vi "auto_direct_attack_v2.vi"() -> ()   [LabVIEW 2012, in "MainProject.lvrbt"]
uses:
  MainProject.lvrbt
  <vilib>/NXT/Hardware/Plugins/Tetrix DC Motor/TetrixDCMotorAddress.ctl
  Drivers/AutoControlDirectAttackV2.ctl
  Drivers/LineDetectCtl.ctl
  Drivers/AutoDriverControl.ctl
  <vilib>/NXT/HiTechnic/HiTechnic Controls/HiTechnic Port.ctl
  <vilib>/NXT/Block Support/NXT_InputPort.ctl
  Drivers/LineCounterControl.ctl
  FTC 2012 - 2013/Controls/SpeedControl.ctl
  <vilib>/NXT/NXTIO Xnodes/NXTIONodeSubVIs/TETRIX IO Check Battery.vi
  <vilib>/NXT/Dual Mode Library/Waits/Wait_Num(msec).vi
  <vilib>/NXT/NXTIO Xnodes/NXTIONodeSubVIs/TETRIX IO Stop DC Motors.vi
  <vilib>/NXT/Dual Mode Library/Sound/Tone.vi
  <vilib>/NXT/Dual Mode Library/Display/drawNumber.vi
  <vilib>/NXT/Subs/LVHSConnector.ctl
  <vilib>/NXT/NXTIO Xnodes/AddressXNode/NXTIOAddress.xnode
  <vilib>/NXT/NXTIO Xnodes/NXTIOXNode/NXTIO.xnode
  <vilib>/NXT/LegoClasses/BrickReference/BrickReference.lvclass
panel:
  out "Enabled":bool
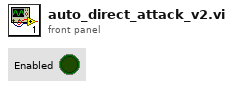
[diagram p1: front panel]
types:
  T1 = typedef "LVHSConnector.ctl" = refnum<class "BrickReference.lvclass">
  T2 = typedef "TetrixDCMotorAddress.ctl" = i16
  T3 = typedef "LineCounterControl.ctl" = enum16{"Reset", "Check"}
  T4 = typedef "HiTechnic Port.ctl" = cluster{"Port":T5, "MUX Port":u8}
  T5 = typedef "NXT_InputPort.ctl" = u8
  T6 = typedef "AutoDriverControl.ctl" = enum16{"Init", "Forward", "Reverse", "Left", "Right", "Brake"}
  T7 = typedef "LineDetectCtl.ctl" = enum16{"Init", "Found?", "Close"}
  T8 = typedef "AutoControlDirectAttackV2.ctl" = enum16{"DecideSide", "Approach", "Align", "DriveToCrate", "DropBlock", "ToEndCrates", "DriveToLine", "TurnAndPark"}
  T9 = typedef "SpeedControl.ctl" = enum16{"Fast", "Medium", "Slow"}
  T10 = cluster{"TetrixDCMotor":T2, "TetrixDCMotor 2":T2}
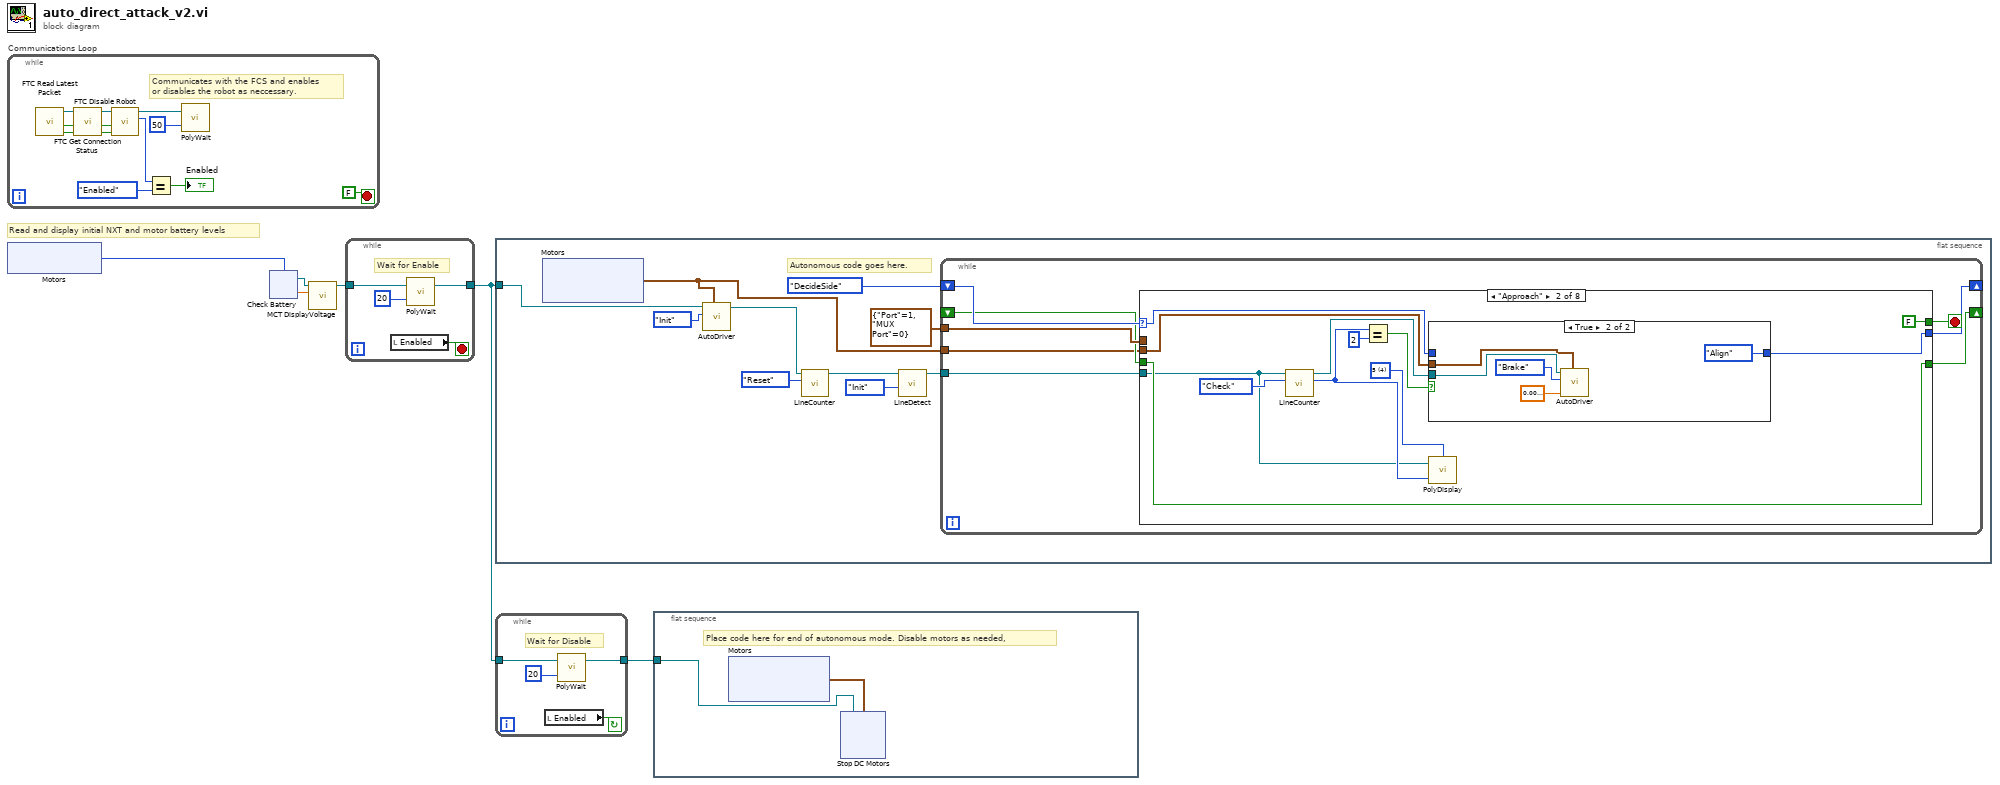
[diagram p0: block diagram]
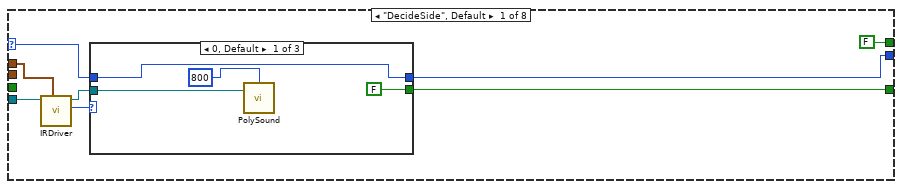
[diagram p2: hidden frame]
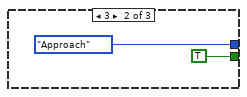
[diagram p3: hidden frame]
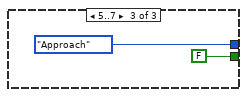
[diagram p4: hidden frame]
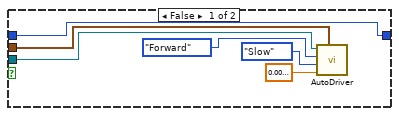
[diagram p5: hidden frame]
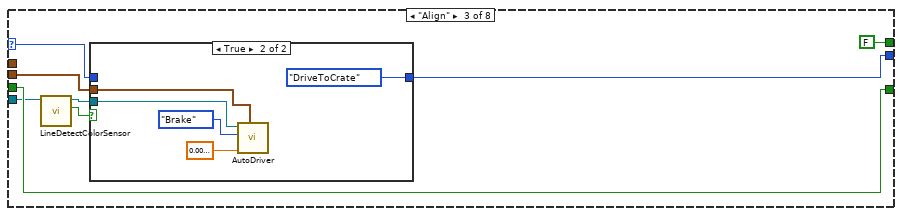
[diagram p6: hidden frame]
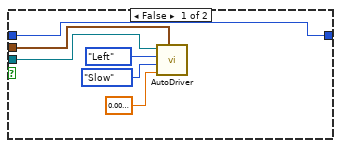
[diagram p7: hidden frame]
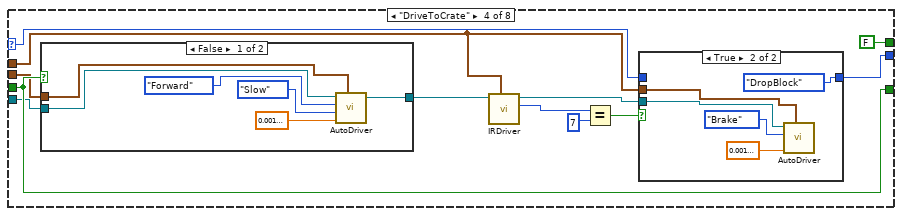
[diagram p8: hidden frame]
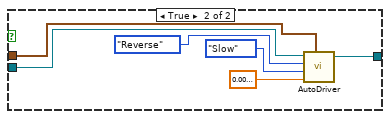
[diagram p10: hidden frame]
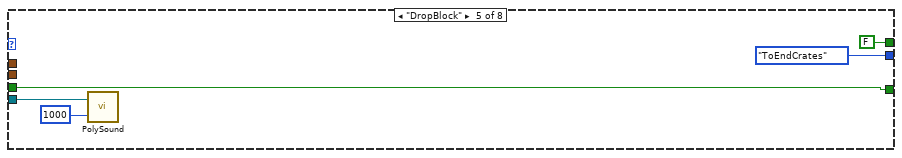
[diagram p11: hidden frame]
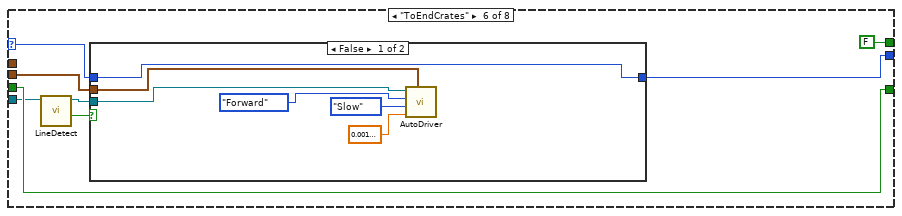
[diagram p12: hidden frame]
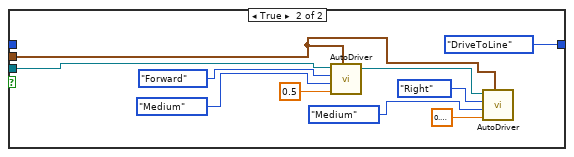
[diagram p13: hidden frame]
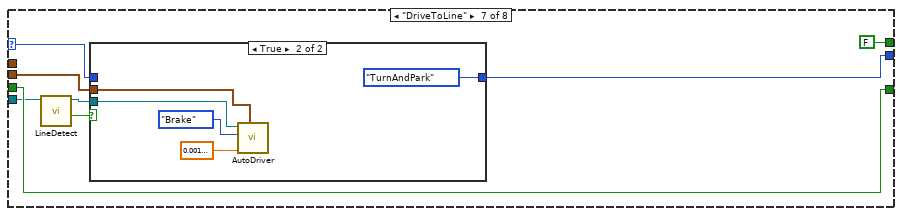
[diagram p14: hidden frame]
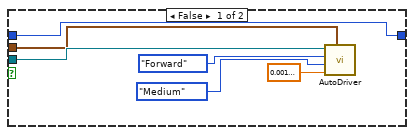
[diagram p15: hidden frame]
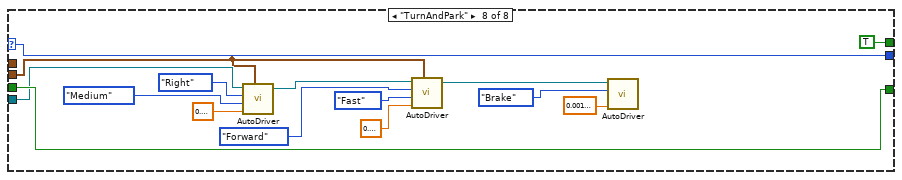
[diagram p16: hidden frame]
diagram:
  # "Read and display initial NXT and motor battery levels"
  n1 = while "Communications Loop" {
    stop <- FALSE stop-if-true
    # "Communicates with the FCS and enables \nor disables the robot as neccessary."
    n2 = call <vilib>:"FTC Read Latest Packet.vi"() -> ("Packet Received?"=w16:bool, "Stopped?"=w15:bool, "NXT"=w18:T1)  [unwired: 6 in, 3 out]
    n3 = call <vilib>:"FTC Get Connection Status.vi"("Packet Received?"=w16, "Stopped?"=w15, "NXT"=w18) -> ("Online?"=w7:bool, "Stopped?"=w8:bool, "NXT"=w17:T1)  [unwired: 5 in]
    n4 = call <vilib>:"FTC Disable Robot.vi"("Online?"=w7, "Stopped?"=w8, "NXT"=w17) -> ("Enabled?"=w11:enum16{"Disabled", "Enabled"}, "NXT"=w13:T1)  [unwired: 3 in]
    n5 = Equal?(x=w11, y=enum16{"Disabled", "Enabled"}."Enabled") -> (x = y?=→"Enabled":bool)
    n6 = call-poly <vilib>:"PolyWait.vi"("Time (100 msec)"=u32 50 ("Time (msec)"), "NXT"=w13) -> ()  [unwired: 2 in, 1 out]
  }
  n7 = xnode "Motors"() -> ("Motor"=w1:T2)
  n8 = xnode "Check Battery"("Motors"=w1) -> ("Voltage 1"=w2:sgl, "NXT"=w4:T1)  [unwired: 1 in]
  n9 = call <vilib>:"MCT DisplayVoltage.vi"("Motor Voltage"=w2, "NXT"=w4) -> ("NXT"=w3:T1)  [unwired: 9 in]
  n10 = while {
    tunnel: [w20] -> w6
    tunnel: w3 -> [w19]
    stop <- w21 stop-if-true
    # "Wait for Enable"
    n11 = local read "Enabled"() -> (w21:bool)
    n12 = call-poly <vilib>:"PolyWait.vi"("Time (100 msec)"=u32 20 ("Time (msec)"), "NXT"=w19) -> ("NXT"=w20:T1)  [unwired: 2 in]
  }
  n13 = flat-sequence {
    tunnel: w6 -> [w31]
    frame #0 {
      # "Autonomous code goes here."
      n14 = xnode "Motors"() -> ("Motor"=w26:cluster{"TetrixDCMotor":T2, "TetrixDCMotor":T2})
      n15 = call "AutoDriver.vi"("NXT In"=w31, "Motors"=w26, "Direction"=AutoDriverControl."Init") -> ("NXT Out"=w25:T1)  [unwired: 5 in]
      n16 = call "LineCounter.vi"("Mode"=LineCounterControl."Reset", "NXT In"=w25) -> ("NXT Out"=w24:T1)  [unwired: 8 in, 1 out]
      n17 = call "LineDetect.vi"("Mode"=LineDetectCtl."Init", "NXT In"=w24) -> ("NXT Out"=w28:T1)  [unwired: 6 in, 1 out]
      n18 = while {
        tunnel: w28 -> [w39]
        tunnel: T4 {"Port"=1, "MUX Port"=0} ("Port") -> [w38]
        shift-right: [w37] -> _
        shift-left: _ -> [w36]
        tunnel: w26 -> [w35]
        shift-right: [w33] -> _
        shift-left: AutoControlDirectAttackV2."DecideSide" -> [w40]
        stop <- w34 stop-if-true
        n19 = case shown="\"Approach\"" w40 {
          selector: w40 -> [w42 w67 w85 w103 _ w136 w160 w177]
          tunnel: w39 -> [w48 w57 w82 w108 w132 w140 w164 w188]
          tunnel: w38 -> [w47 _ _ w100 _ _ _ _]
          tunnel: [w45 w68 w87 w110 w133 w141 w165 w191] -> w37
          tunnel: w36 -> [_ w68 w87 w110 w133 w141 w165 w191]
          tunnel: [w44 w65 w84 w102 AutoControlDirectAttackV2."ToEndCrates" w135 w159 w177] -> w33
          tunnel: w35 -> [_ w66 w86 w109 _ w137 w161 w184]
          tunnel: [FALSE FALSE FALSE FALSE FALSE FALSE FALSE TRUE] -> w34
          frame "DecideSide", Default {
            n20 = call "IRDriver.vi"("Port"=w47, "NXT In"=w48) -> ("Sector (0-9)"=w46:i16, "NXT Out"=w43:T1)  [unwired: 8 in]
            n21 = case shown="0, Default" w46 {
              tunnel: [FALSE TRUE FALSE] -> w45
              tunnel: [w49 AutoControlDirectAttackV2."Approach" AutoControlDirectAttackV2."Approach"] -> w44
              tunnel: w43 -> [w51 _ _]
              tunnel: w42 -> [w49 _ _]
              frame 0, Default {
                n22 = call-poly <vilib>:"PolySound.vi"("NXT"=w51, "Tone (440 Hz)"=u16 800) -> ()  [unwired: 2 in, 1 out]
              }
              frame 3 {
              }
              frame 5..7 {
              }
            }
          }
          frame "Approach" {
            w58 = i16 4 items=["1", "2", "3", "4", "5", "6", "7", "8"] ("Line")
            n23 = call "LineCounter.vi"("Mode"=LineCounterControl."Check", "NXT In"=w57) -> ("NumOfLines"=w59:i32, "NXT Out"=w63:T1)  [unwired: 8 in]
            n24 = Equal?(x=w59, y=2) -> (x = y?=w60:bool)
            n25 = case shown="True" w60 {
              tunnel: w67 -> [w72 _]
              tunnel: w63 -> [w74 w79]
              tunnel: w66 -> [w73 w77]
              tunnel: [w72 AutoControlDirectAttackV2."Align"] -> w65
              frame False {
                n26 = call "AutoDriver.vi"("NXT In"=w74, "Motors"=w73, "Direction"=AutoDriverControl."Forward", "Speed"=SpeedControl."Slow", "Time (1 sec)"=sgl 0.01) -> ()  [unwired: 3 in, 1 out]
              }
              frame True {
                n27 = call "AutoDriver.vi"("NXT In"=w79, "Motors"=w77, "Direction"=AutoDriverControl."Brake", "Time (1 sec)"=sgl 0.01) -> ()  [unwired: 4 in, 1 out]
              }
            }
            n28 = call-poly <vilib>:"PolyDisplay.vi"("number"=w59, "NXT"=w57, "Line"=w58) -> ()  [unwired: 1 in, 1 out]
          }
          frame "Align" {
            n29 = call "LineDetectColorSensor.vi"("NXT In"=w82) -> ("CrossedLine?"=w81:bool, "NXT Out"=w80:T1)  [unwired: 9 in]
            n30 = case shown="True" w81 {
              tunnel: w80 -> [w93 w98]
              tunnel: w86 -> [w92 w97]
              tunnel: w85 -> [w88 _]
              tunnel: [w88 AutoControlDirectAttackV2."DriveToCrate"] -> w84
              frame False {
                n31 = call "AutoDriver.vi"("NXT In"=w93, "Motors"=w92, "Direction"=AutoDriverControl."Left", "Speed"=SpeedControl."Slow", "Time (1 sec)"=sgl 0.01) -> ()  [unwired: 3 in, 1 out]
              }
              frame True {
                n32 = call "AutoDriver.vi"("NXT In"=w98, "Motors"=w97, "Direction"=AutoDriverControl."Brake", "Time (1 sec)"=sgl 0.01) -> ()  [unwired: 4 in, 1 out]
              }
            }
          }
          frame "DriveToCrate" {
            n33 = case shown="False" w110 {
              tunnel: w108 -> [w118 w128]
              tunnel: w109 -> [w119 w127]
              tunnel: [w117 w123] -> w107
              frame False {
                n34 = call "AutoDriver.vi"("NXT In"=w118, "Motors"=w119, "Direction"=AutoDriverControl."Forward", "Speed"=SpeedControl."Slow", "Time (1 sec)"=sgl 0.001) -> ("NXT Out"=w117:T1)  [unwired: 3 in]
              }
              frame True {
                n35 = call "AutoDriver.vi"("NXT In"=w128, "Motors"=w127, "Direction"=AutoDriverControl."Reverse", "Speed"=SpeedControl."Slow", "Time (1 sec)"=sgl 0.01) -> ("NXT Out"=w123:T1)  [unwired: 3 in]
              }
            }
            n36 = call "IRDriver.vi"("Port"=w100, "NXT In"=w107) -> ("Sector (0-9)"=w106:i16, "NXT Out"=w101:T1)  [unwired: 8 in]
            n37 = Equal?(x=w106, y=i16 7) -> (x = y?=w104:bool)
            n38 = case shown="True" w104 {
              tunnel: w103 -> [w111 _]
              tunnel: [w111 AutoControlDirectAttackV2."DropBlock"] -> w102
              tunnel: w101 -> [_ w115]
              tunnel: w100 -> [_ w114]
              frame False {
              }
              frame True {
                n39 = call "AutoDriver.vi"("NXT In"=w115, "Motors"=w114, "Direction"=AutoDriverControl."Brake", "Time (1 sec)"=sgl 0.001) -> ()  [unwired: 4 in, 1 out]
              }
            }
          }
          frame "DropBlock" {
            n40 = call-poly <vilib>:"PolySound.vi"("Duration (500 ms)"=u16 1000, "NXT"=w132) -> ()  [unwired: 2 in, 1 out]
          }
          frame "ToEndCrates" {
            n41 = call "LineDetect.vi"("NXT In"=w140) -> ("Line Found?"=w139:bool, "NXT Out"=w138:T1)  [unwired: 7 in]
            n42 = case shown="False" w139 {
              tunnel: w138 -> [w146 w157]
              tunnel: w137 -> [w145 w152]
              tunnel: w136 -> [w147 _]
              tunnel: [w147 AutoControlDirectAttackV2."DriveToLine"] -> w135
              frame False {
                n43 = call "AutoDriver.vi"("NXT In"=w146, "Motors"=w145, "Direction"=AutoDriverControl."Forward", "Speed"=SpeedControl."Slow", "Time (1 sec)"=sgl 0.001) -> ()  [unwired: 3 in, 1 out]
              }
              frame True {
                n44 = call "AutoDriver.vi"("NXT In"=w157, "Motors"=w152, "Direction"=AutoDriverControl."Forward", "Speed"=SpeedControl."Medium", "Time (1 sec)"=sgl 0.5) -> ("NXT Out"=w153:T1)  [unwired: 3 in]
                n45 = call "AutoDriver.vi"("NXT In"=w153, "Motors"=w152, "Direction"=AutoDriverControl."Right", "Speed"=SpeedControl."Medium", "Time (1 sec)"=sgl 0.8) -> ()  [unwired: 3 in, 1 out]
              }
            }
          }
          frame "DriveToLine" {
            n46 = call "LineDetect.vi"("NXT In"=w164) -> ("Line Found?"=w163:bool, "NXT Out"=w162:T1)  [unwired: 7 in]
            n47 = case shown="True" w163 {
              tunnel: w162 -> [w171 w175]
              tunnel: w161 -> [w170 w176]
              tunnel: w160 -> [w166 _]
              tunnel: [w166 AutoControlDirectAttackV2."TurnAndPark"] -> w159
              frame False {
                n48 = call "AutoDriver.vi"("NXT In"=w171, "Motors"=w170, "Direction"=AutoDriverControl."Forward", "Speed"=SpeedControl."Medium", "Time (1 sec)"=sgl 0.001) -> ()  [unwired: 3 in, 1 out]
              }
              frame True {
                n49 = call "AutoDriver.vi"("NXT In"=w175, "Motors"=w176, "Direction"=AutoDriverControl."Brake", "Time (1 sec)"=sgl 0.001) -> ()  [unwired: 4 in, 1 out]
              }
            }
          }
          frame "TurnAndPark" {
            n50 = call "AutoDriver.vi"("NXT In"=w188, "Motors"=w184, "Direction"=AutoDriverControl."Right", "Speed"=SpeedControl."Medium", "Time (1 sec)"=sgl 0.8) -> ("NXT Out"=w185:T1)  [unwired: 3 in]
            n51 = call "AutoDriver.vi"("NXT In"=w185, "Motors"=w184, "Direction"=AutoDriverControl."Forward", "Speed"=SpeedControl."Fast", "Time (1 sec)"=sgl 0.7) -> ("NXT Out"=w180:T1)  [unwired: 3 in]
            n52 = call "AutoDriver.vi"("NXT In"=w180, "Direction"=AutoDriverControl."Brake", "Time (1 sec)"=sgl 0.001) -> ()  [unwired: 5 in, 1 out]
          }
        }
      }
    }
  }
  n53 = while {
    tunnel: [w194] -> w5
    tunnel: w6 -> [w193]
    stop <- w195 continue-if-true
    # "Wait for Disable"
    n54 = local read "Enabled"() -> (w195:bool)
    n55 = call-poly <vilib>:"PolyWait.vi"("Time (100 msec)"=u32 20 ("Time (msec)"), "NXT"=w193) -> ("NXT"=w194:T1)  [unwired: 2 in]
  }
  n56 = flat-sequence {
    tunnel: w5 -> [w198]
    frame #0 {
      # "Place code here for end of autonomous mode. Disable motors as needed,"
      n57 = xnode "Motors"() -> ("Motor"=w197:cluster{"TetrixDCMotor":T2, "TetrixDCMotor":T2})
      n58 = xnode "Stop DC Motors"("Motors"=w197, "NXT"=w198) -> ()  [unwired: 1 out]
    }
  }
